vi "axis_Grab.vi"(10 "stop":bool, 11 "address":string="192.168.1.200") -> (3 "Image":T2(plugin-control))   [LabVIEW 2009]
doc: "Field of View of Axis 207\nWidth 106 degree\nHeight 74 degree"
panel:
  in  "Color?":bool=TRUE
  in  "Pixel Format":T1(ring)=enum."640 x 480 MJPG"
  out "error out":errorcluster={"status"=TRUE, "code"=-1074396120, "source"="IMAQ ReadFile\n  Not an image."}
  out "Content Length":i32=37577
  in  "Frame Rate":u32(slide) max=30 scale=0.0..30.0
  in  "Compression":u32(slide)=25 scale=0.0..99.0
  # "Field of View\n106 degree width\n74 degree height"
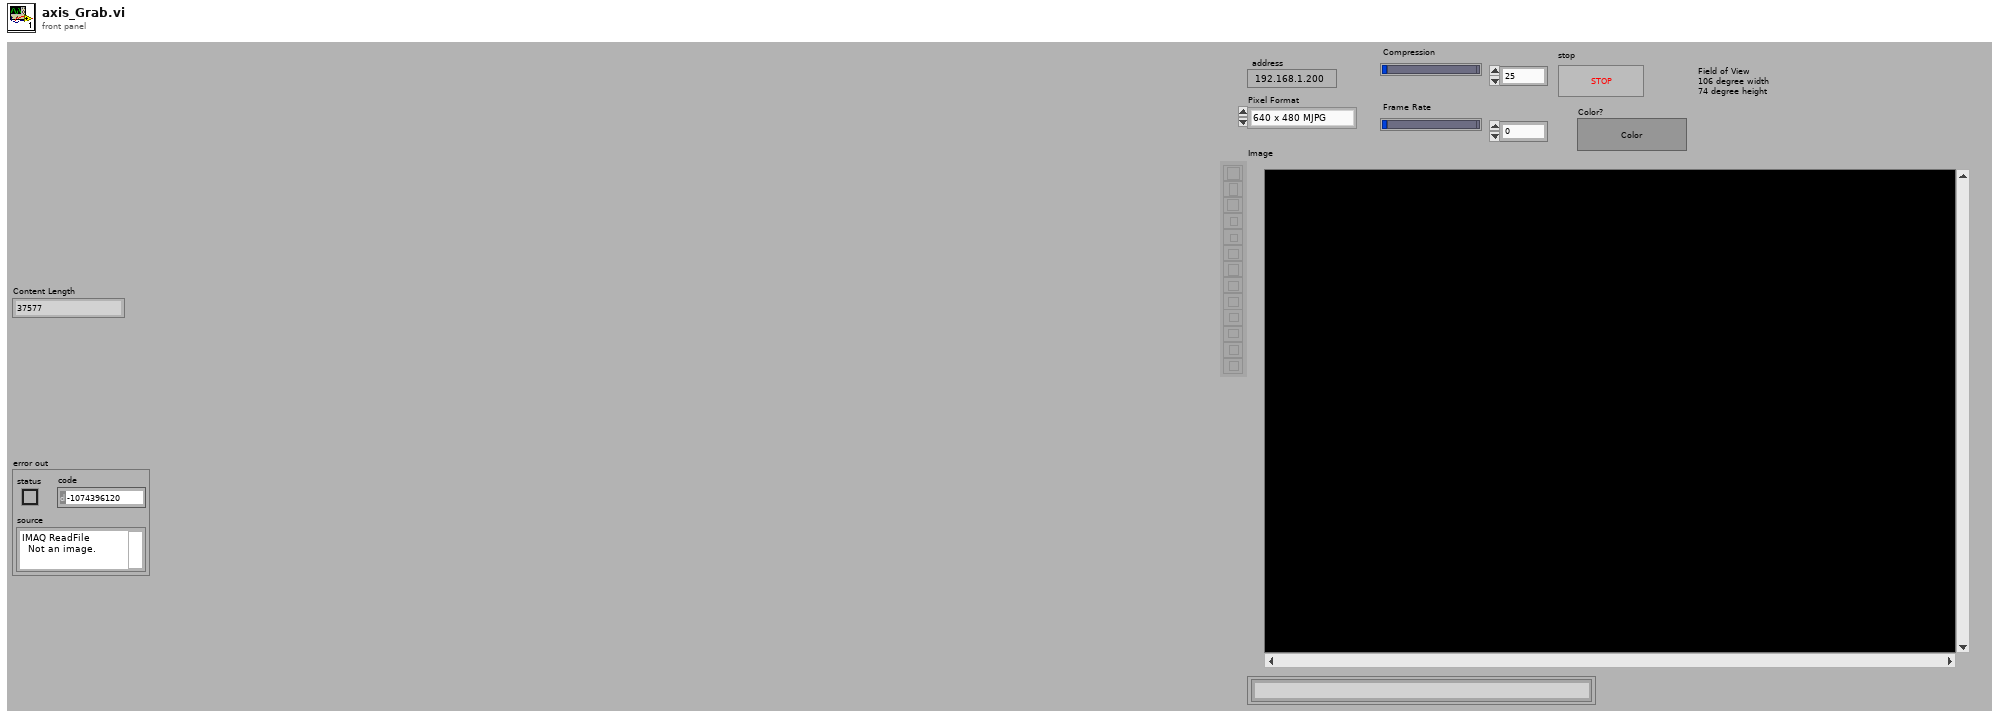
[diagram p1: front panel]
types:
  T1 = enum16{"1280 x 1024 MJPG", "1280 x 960 MJPG", "1280 x 720 MJPG", "1280 x 480 MJPG", "640 x 480 MJPG", "320 x 240 MJPG", "160 x 120 MJPG"}
  T2 = typedef "IMAQ Image.ctl" = refnum<image>
  T3 = enum16{"Standard", "Buffered", "CRLF", "Immediate"}
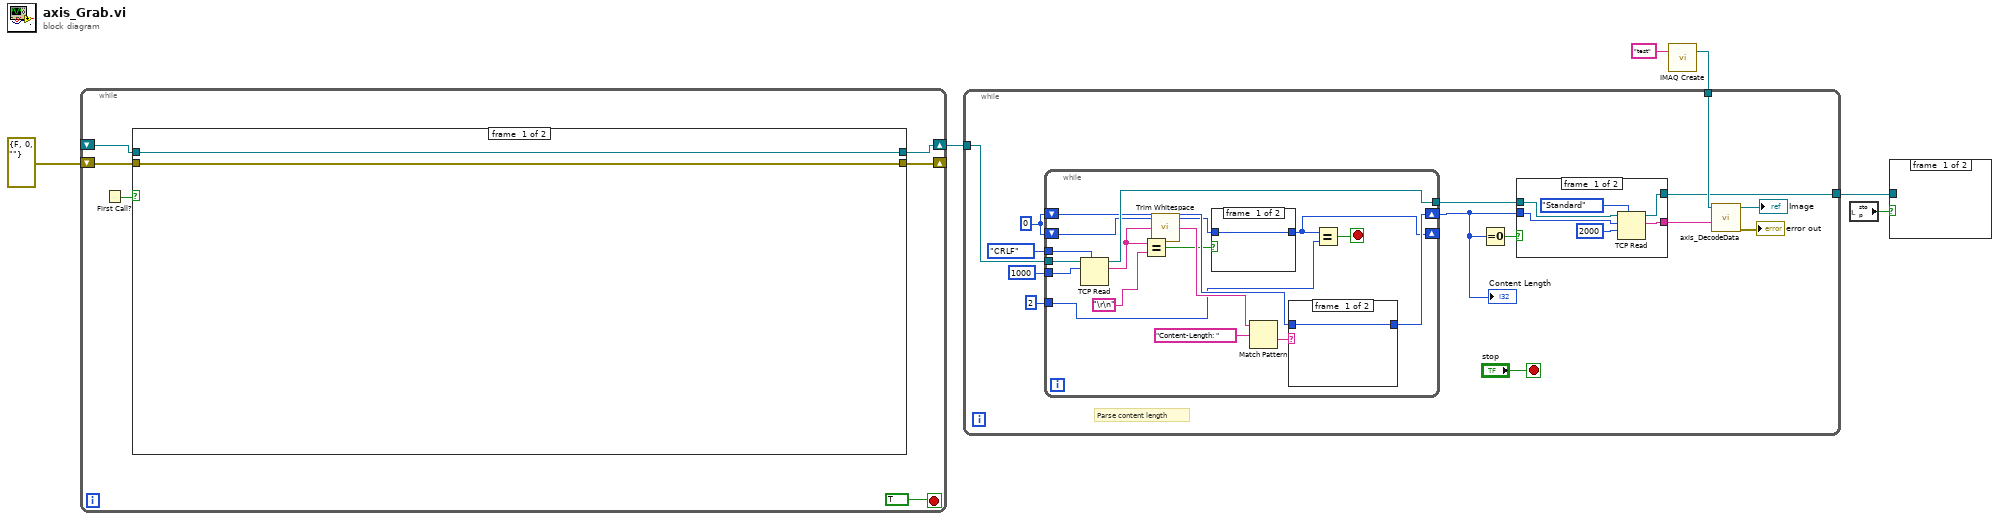
[diagram p0: block diagram]
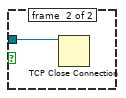
[diagram p2: hidden frame]
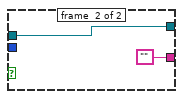
[diagram p3: hidden frame]
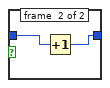
[diagram p4: hidden frame]
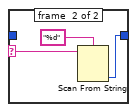
[diagram p5: hidden frame]
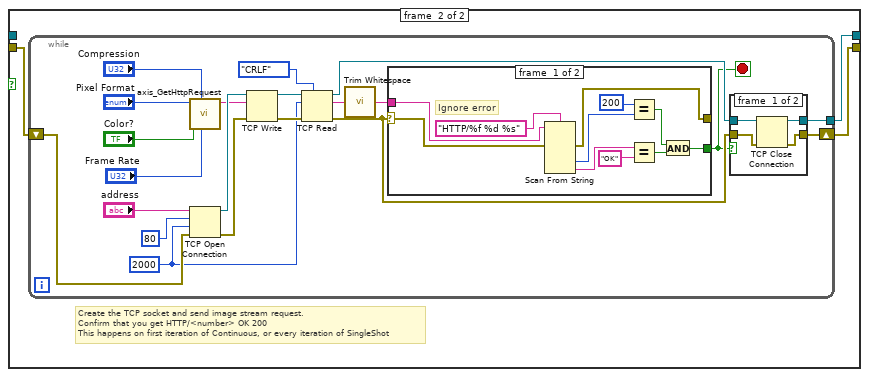
[diagram p6: hidden frame]
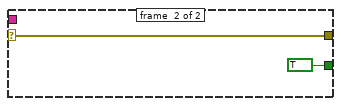
[diagram p8: hidden frame]
diagram:
  n1 = while {
    shift-right: [w9] -> w4
    shift-left: _ -> [w8]
    shift-right: [w10] -> _
    shift-left: errorcluster {"status"=FALSE, "code"=0, "source"=""} ("error out") -> [w11]
    stop <- TRUE stop-if-true
    n2 = First Call?() -> (First Call?: T/F=w7:bool)
    n3 = case shown="True" w7 {
      tunnel: w11 -> [w13 w17]
      tunnel: [w13 w16] -> w10
      tunnel: [w14 w15] -> w9
      tunnel: w8 -> [w14 _]
      frame #0 {
      }
      frame #1 {
        # "Create the TCP socket and send image stream request.\nConfirm that you get HTTP/<number> OK 200\nThis happens on first iteration of Continuous, or every iteration of SingleShot"
        n4 = while {
          shift-right: [w26] -> w16
          shift-left: w17 -> [w31]
          tunnel: [w27] -> w15
          stop <- w25 stop-if-true
          w18 = 2000 ("timeout ms (60000)")
          n5 = call "axis_GetHttpRequest.vi"("Frame Rate"="Frame Rate", "Compression"="Compression", "Color?"="Color?", "Pixel Format"="Pixel Format") -> ("HTTP Request"=w24:string)  [unwired: 7 out]
          n6 = TCP Open Connection(address="address", remote port or service name=u16 80, timeout ms (60000)=w18, error in (no error)=w31) -> (connection ID=w32:refnum<k5>, error out=w30:errorcluster)  [unwired: 1 out]
          n7 = TCP Write(connection ID=w32, data in=w24, error in (no error)=w30) -> (connection ID out=w35:refnum<k5>, error out=w34:errorcluster)  [unwired: 2 out]
          n8 = TCP Read(connection ID=w35, bytes to read=w18, error in (no error)=w34, 7:T3."CRLF" ("mode (standard)")) -> (connection ID out=w29:refnum<k5>, data out=w38:string, error out=w28:errorcluster)  [unwired: 1 out]
          n9 = call <vilib>:"Trim Whitespace.vi"("string"=w38) -> ("trimmed string"=w36:string)  [unwired: 1 in]
          n10 = case shown="No Error" w28 {
            selector: w28 -> [w46 w57]
            tunnel: w36 -> [w55 _]
            tunnel: [w47 TRUE] -> w25
            tunnel: [w45 w57] -> _
            frame #0 {
              # "Ignore error"
              n11 = Scan From String(format string="HTTP/%f %d %s", input string=w55, error in=w46) -> (error out=w45:errorcluster, output 2=w53:i32, output 3=w51:string)  [unwired: 1 in, 6 out]
              n12 = Equal?(x=200, y=w53) -> (x = y?=w48:bool)
              n13 = Equal?(x=w51, y="OK" ("format string")) -> (x = y?=w49:bool)
              n14 = And(x=w48, y=w49) -> (x .and. y?=w47:bool)
            }
            frame #1 {
            }
          }
          n15 = case shown="False" w25 {
            tunnel: w29 -> [w42 w44]
            tunnel: w28 -> [w41 w43]
            tunnel: [w40 w44] -> w27
            tunnel: [w39 w43] -> w26
            frame #0 {
              n16 = TCP Close Connection(connection ID=w42, error in (no error)=w41) -> (connection ID out=w40:refnum<k5>, error out=w39:errorcluster)  [unwired: 1 out]
            }
            frame #1 {
            }
          }
        }
      }
    }
  }
  n17 = call "IMAQ Create"("Image Name"="test") -> ("New Image"=w3:T2)  [unwired: 3 in, 2 out]
  n18 = while {
    tunnel: w4 -> [w71]
    tunnel: w3 -> [w68]
    tunnel: [w65] -> w2
    stop <- "stop" stop-if-true
    w64 = 0
    # "Parse content length"
    n19 = while {
      tunnel: [w95] -> w59
      shift-right: [w91] -> w62
      shift-left: w64 -> [w90]
      shift-right: [w87] -> _
      shift-left: w64 -> [w88]
      tunnel: 1000 ("bytes to read") -> [w85]
      tunnel: T3."CRLF" ("mode (standard)") -> [w84]
      tunnel: w71 -> [w83]
      tunnel: 2 ("y") -> [w82]
      stop <- w80 stop-if-true
      n20 = TCP Read(connection ID=w83, bytes to read=w85, 7:w84) -> (connection ID out=w95:refnum<k5>, data out=w86:string)  [unwired: 1 in, 2 out]
      n21 = Equal?(x=w86, y="\r\n") -> (x = y?=w89:bool)
      n22 = call <vilib>:"Trim Whitespace.vi"("string"=w86) -> ("trimmed string"=w93:string)  [unwired: 1 in]
      n23 = case shown="True" w89 {
        tunnel: w88 -> [w96 w98]
        tunnel: [w96 w97] -> w87
        frame #0 {
        }
        frame #1 {
          n24 = Increment(x=w98) -> (x+1=w97:i32)
        }
      }
      n25 = Match Pattern(string=w93, regular expression="Content-Length: ") -> (after substring=w92:string)  [unwired: 4 out]
      n26 = case shown="\"True\", Default" w92 {
        selector: w92 -> [_ w101]
        tunnel: [w99 w102] -> w91
        tunnel: w90 -> [w99 _]
        frame #0 {
        }
        frame #1 {
          n27 = Scan From String(format string="%d", input string=w101) -> (output 1=w102:i32)  [unwired: 2 in, 4 out]
        }
      }
      n28 = Equal?(x=w87, y=w82) -> (x = y?=w80:bool)
    }
    "Content Length" <- w62
    n29 = Equal To 0?(x=w62) -> (x = 0?=w63:bool)
    n30 = case shown="False" w63 {
      tunnel: w59 -> [w77 w78]
      tunnel: [w73 ""] -> w67
      tunnel: w62 -> [w74 _]
      tunnel: [w72 w78] -> w65
      frame #0 {
        n31 = TCP Read(connection ID=w77, bytes to read=w74, 7:T3."Standard" ("mode (standard)"), 9:2000 ("timeout ms (25000)")) -> (connection ID out=w72:refnum<k5>, data out=w73:string)  [unwired: 1 in, 1 out]
      }
      frame #1 {
      }
    }
    n32 = call "axis_DecodeData.vi"("Data In"=w67, "Image In"=w68) -> ("error out"=→"error out":errorcluster, "Image Out"=→"Image":T2)  [unwired: 2 in, 6 out]
  }
  n33 = local read "stop"() -> (w1:bool)
  n34 = case shown="True" w1 {
    tunnel: w2 -> [_ w103]
    frame #0 {
    }
    frame #1 {
      n35 = TCP Close Connection(connection ID=w103) -> ()  [unwired: 2 in, 2 out]
    }
  }
